vi "imagetest.vi"() -> ()   [LabVIEW 2015]
uses:
  <vilib>/vision/NI_Vision_Development_Module.lvlib
panel:
  out "Image Type":T1 items=["Grayscale (U8)", "Grayscale (I16)", "Grayscale (SGL)", "Complex (CSG)", "RGB (U32)", "HSL (U32)", "RGB (U64)", "Grayscale (U16)"]
  out "Image 3":T2(plugin-control)
  out "Image 2":T2(plugin-control)
  out "File Type out":string
  out "Image":T2(plugin-control)
  out "error out":errorcluster
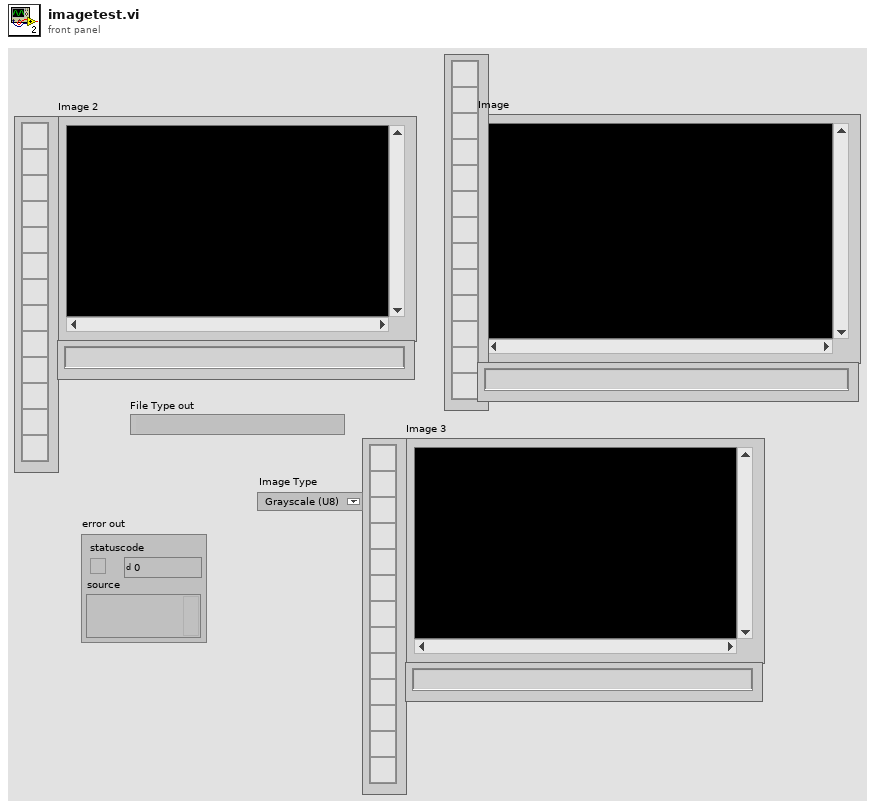
[diagram p1: front panel]
types:
  T1 = typedef "Image Type" = u32
  T2 = typedef "IMAQ Image.ctl" = refnum<image>
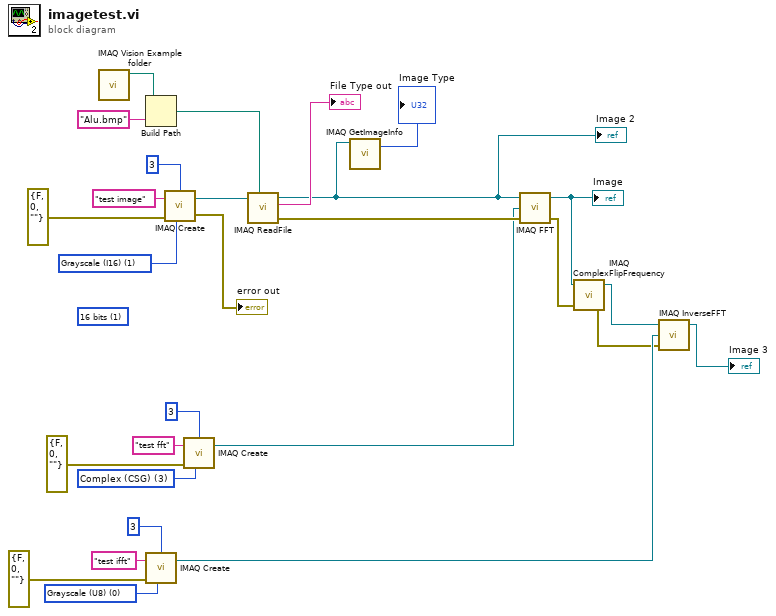
[diagram p0: block diagram]
diagram:
  w8 = T1 0 items=["Grayscale (U8)", "Grayscale (I16)", "Grayscale (SGL)", "Complex (CSG)", "RGB (U32)", "HSL (U32)", "RGB (U64)", "Grayscale (U16)"] ("Image Type")
  (unwired) u32 1 items=["8 bits", "16 bits", "Float", "Complex", "RGB", "HSL"] ("Image Type")
  w15 = T1 3 items=["Grayscale (U8)", "Grayscale (I16)", "Grayscale (SGL)", "Complex (CSG)", "RGB (U32)", "HSL (U32)", "RGB (U64)", "Grayscale (U16)"] ("Image Type")
  w14 = T1 1 items=["Grayscale (U8)", "Grayscale (I16)", "Grayscale (SGL)", "Complex (CSG)", "RGB (U32)", "HSL (U32)", "RGB (U64)", "Grayscale (U16)"] ("Image Type")
  n1 = call "IMAQ Vision Example folder.vi"() -> ("Example Image Path"=w24:path)  [unwired: 11 in]
  n2 = Build Path(base path=w24, name or relative path="Alu.bmp") -> (appended path=w21:path)
  n3 = call "IMAQ Create"("Border Size"=3, "Image Name"="test ifft", "Image Type"=w8, "error in (no error)"=errorcluster {"status"=FALSE, "code"=0, "source"=""}) -> ("New Image"=w7:T2)  [unwired: 1 in, 1 out]
  n4 = call "IMAQ Create"("Border Size"=3, "Image Name"="test image", "Image Type"=w14, "error in (no error)"=errorcluster {"status"=FALSE, "code"=0, "source"=""}) -> ("New Image"=w22:T2, "error out"=→"error out":errorcluster)  [unwired: 1 in]
  n5 = call "IMAQ Create"("Border Size"=3, "Image Name"="test fft", "Image Type"=w15, "error in (no error)"=errorcluster {"status"=FALSE, "code"=0, "source"=""}) -> ("New Image"=w13:T2)  [unwired: 1 in, 1 out]
  n6 = call "IMAQ ReadFile"("File Path"=w21, "Image"=w22) -> ("error out"=w16:errorcluster, "File Type out"=→"File Type out":string, "Image Out"=w2:T2)  [unwired: 5 in, 2 out]
  "Image 2" <- w2
  n7 = call "IMAQ GetImageInfo"("Image"=w2) -> ("Image Type"=→"Image Type":T1)  [unwired: 3 in, 7 out]
  n8 = call "IMAQ FFT"("error in (no error)"=w16, "Image Dst"=w13, "Image Src"=w2) -> ("error out"=w4:errorcluster, "Image Dst Out"=w6:T2)  [unwired: 1 in]
  "Image" <- w6
  n9 = call "IMAQ ComplexFlipFrequency"("error in (no error)"=w4, "Image Src"=w6) -> ("error out"=w3:errorcluster, "Image Dst Out"=w5:T2)  [unwired: 2 in]
  n10 = call "IMAQ InverseFFT"("error in (no error)"=w3, "Image Dst"=w7, "Image Src"=w5) -> ("Image Dst Out"=→"Image 3":T2)  [unwired: 1 in, 1 out]
